vi "iWorx Get Visible Chart Data.vi"(7 "Selection Chart":refnum<vi>, 8 "Error In":errorcluster) -> (0 "Error Out":errorcluster, 2 "Waveform out":waveform(dbl), 4 "Y Length":i32)   [LabVIEW 2012]
uses:
  <vilib>/Waveform/WDTOps.llb/WDT Append Waveforms DBL.vi
  <vilib>/Waveform/WDTOps.llb/WDT Get Waveform Subset DBL.vi
panel:
  out "Time":dbl
  out "Portion":dbl
  out "size(s)":i32
  out "t0":timestamp
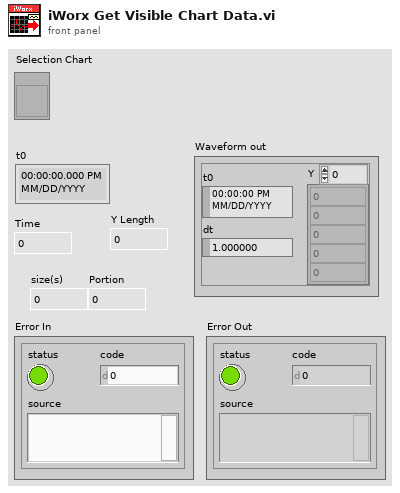
[diagram p1: front panel]
types:
  T1 = typedef "LVRangeTypeDef.ctl" = cluster{"Minimum":dbl, "Maximum":dbl, "Increment":dbl, "Minor Increment":dbl, "Start":dbl}
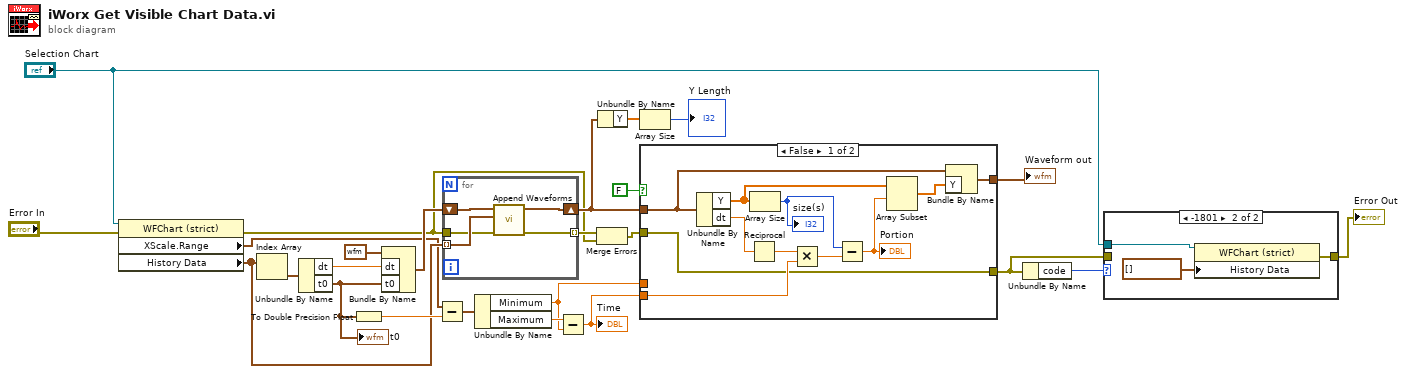
[diagram p0: block diagram]
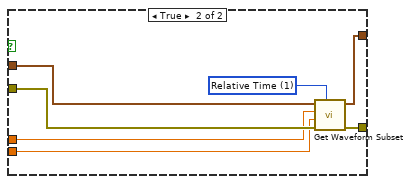
[diagram p2: hidden frame]
diagram:
  n1 = property class="WFChart (strict)"(reference="Selection Chart", error in="Error In") -> (error out=w4:errorcluster, "XScale.Range"=w7:T1, "History Data"=w11:waveform(dbl)[])  [unwired: 1 out]
  n2 = Index Array(array=w11) -> (element=w10:waveform(dbl))  [unwired: 1 in]
  n3 = Unbundle By Name(w10) -> ("dt"=w20:dbl, "t0"=w19:timestamp)
  "t0" <- w19
  n4 = To Double Precision Float(number=w19) -> (double precision float=w17:dbl)
  n5 = Bundle By Name(cluster=waveform(dbl) {"t0"=timestamp(0 s since 1904-01-01), "dt"=2.267573696145e-05, "Y"=[]} ("waveform out"), "dt"=w20, "t0"=w19) -> (w22:waveform(dbl))
  n6 = Subtract(x=w7, y=w17) -> (x-y=w18:T1)
  n7 = for {
    tunnel: w11 -> [w29] mode=indexing
    shift-right: [w30] -> w9
    shift-left: w22 -> [w28]
    tunnel: w4 -> [w27]
    tunnel: [w26] -> w23 mode=indexing
    n8 = call-poly <vilib>:"Append Waveforms.vi"("error in (no error)"=w27, "waveform B"=w29, "waveform A"=w28) -> ("error out"=w26:errorcluster, "waveform out"=w30:waveform(dbl))  [unwired: 7 in]
  }
  n9 = Unbundle By Name(w18) -> ("Minimum"=w8:dbl, "Maximum"=w21:dbl)
  n10 = Subtract(x=w21, y=w8) -> (x-y=w6:dbl)
  "Time" <- w6
  n11 = Merge Errors(w23, w4) -> (w24:errorcluster)
  n12 = Unbundle By Name(w9) -> ("Y"=w13:dbl[])
  n13 = Array Size(array=w13) -> (size(s)=→"Y Length":i32)
  n14 = case shown="False" FALSE {
    tunnel: w24 -> [w31 w48]
    tunnel: [w31 w46] -> w14
    tunnel: [w32 w45] -> w1
    tunnel: w9 -> [w35 w44]
    tunnel: w8 -> [_ w43]
    tunnel: w6 -> [w40 w42]
    frame False {
      n15 = Unbundle By Name(w35) -> ("Y"=w36:dbl[], "dt"=w38:dbl)
      n16 = Reciprocal(x=w38) -> (1/x=w37:dbl)
      n17 = Array Size(array=w36) -> (size(s)=w41:i32)
      "size(s)" <- w41
      n18 = Multiply(x=w37, y=w40) -> (x*y=w39:dbl)
      n19 = Subtract(x=w41, y=w39) -> (x-y=w33:dbl)
      "Portion" <- w33
      n20 = Array Subset(array=w36, index=w33) -> (w34:dbl[])  [unwired: 1 in]
      n21 = Bundle By Name(cluster=w35, "Y"=w34) -> (w32:waveform(dbl))
    }
    frame True {
      w47 = u16 1 items=["Samples", "Relative Time"] ("start/duration format")
      n22 = call-poly <vilib>:"Get Waveform Subset.vi"("start/duration format"=w47, "error in (no error)"=w48, "duration"=w42, "start samples/time"=w43, "waveform in"=w44) -> ("error out"=w46:errorcluster, "waveform out"=w45:waveform(dbl))  [unwired: 1 in, 2 out]
    }
  }
  "Waveform out" <- w1
  n23 = Unbundle By Name(w14) -> ("code"=w16:i32)
  n24 = case shown="-1801" w16 {
    tunnel: "Selection Chart" -> [_ w51]
    tunnel: w14 -> [w49 _]
    tunnel: [w49 w50] -> w2
    frame 0, Default {
    }
    frame -1801 {
      n25 = property class="WFChart (strict)"(reference=w51, "History Data"=waveform(dbl)[] []) -> (error out=w50:errorcluster)  [unwired: 1 in, 1 out]
    }
  }
  "Error Out" <- w2
